vi "Save Default RT Settings to XML FIles_Core.vi"() -> ()   [LabVIEW 2014]
uses:
  <vilib>/Utility/xml.llb/Write to XML File(string).vi
panel:
  out "error out med":errorcluster
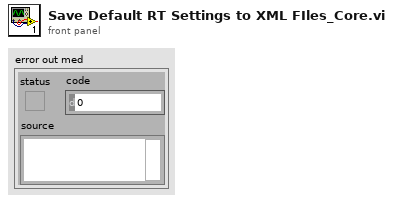
[diagram p1: front panel]
types:
  T1 = typedef "System_Settings_Cluster_dBase_RT_Core.ctl" = cluster{"Units in the system":T2[], "dBase names by units":string[], "dBase User Name_RT":string, "dBase User Password_RT":string, "Number of points to average for stationary state":i32[], "Number of points to collect for saving waveforms per channel":i32[], "Maximum Number of Elements to Keep in dBase Trend History":i32[], "Maximum Number of Waveform Events to Keep in dBase":i32[]}
  T2 = typedef "Unit_Names_Core.ctl" = enum16{"Not used", "Unit 1", "Unit 2", "Unit 3", "Unit 4", "Unit 5", "Unit 6", "Unit 7", "Unit 8", "Unit 9"}
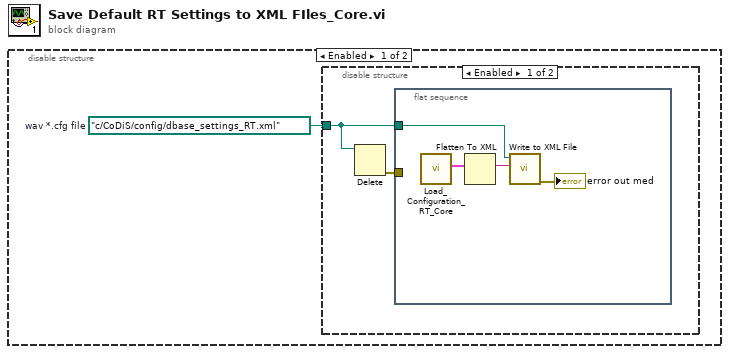
[diagram p0: block diagram]
diagram:
  n1 = disable-structure shown="Enabled" {
    frame Enabled {
      w1 = path "c:/CoDiS/config/dbase_settings_RT.xml"  # wav *.cfg file
      n2 = disable-structure shown="Enabled" {
        disable-tunnel: w1 -> [w3 _]
        frame Enabled {
          n3 = Delete(path (use dialog)=w3) -> (error out=w2:errorcluster)  [unwired: 4 in, 2 out]
          n4 = flat-sequence {
            tunnel: w3 -> [w4]
            tunnel: w2 -> [_]
            frame #0 {
              n5 = call "Load_Configuration_RT_Core.vi"() -> ("System_settings_dBase_RT OUT"=w6:T1)  [unwired: 11 in]
              n6 = Flatten To XML(anything=w6) -> (xml string=w7:string)
              n7 = call-poly <vilib>:"Write to XML File.vi"("XML Input"=w7, "XML File Path"=w4) -> ("error out"=→"error out med":errorcluster)  [unwired: 7 in, 2 out]
            }
          }
        }
        frame Disabled {
        }
      }
    }
    frame Disabled {
    }
  }
